vi "iRobot UART Open.vi"(9 "Baud Rate (BPS)":T1=enum."57600", 11 "UART port in":T2) -> (0 "error out":errorcluster, 3 "UART port out":T2)   [LabVIEW 2010]
doc: "Opens a UART session with an iRobot."
uses:
  UART Port Type.ctl
  Command/Command Controls/iRobot Baud.ctl
  <vilib>/Instr/_visa.llb/VISA Configure Serial Port (Instr).vi
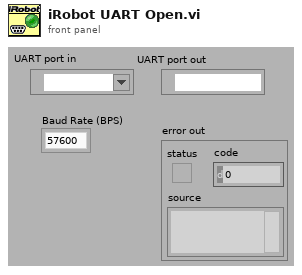
[diagram p1: front panel]
types:
  T1 = typedef "iRobot Baud.ctl" = enum8{"300", "600", "1200", "2400", "4800", "9600", "14400", "19200", "28800", "38400", "57600", "115200"}
  T2 = typedef "UART Port Type.ctl" = refnum<visa-resource-name>
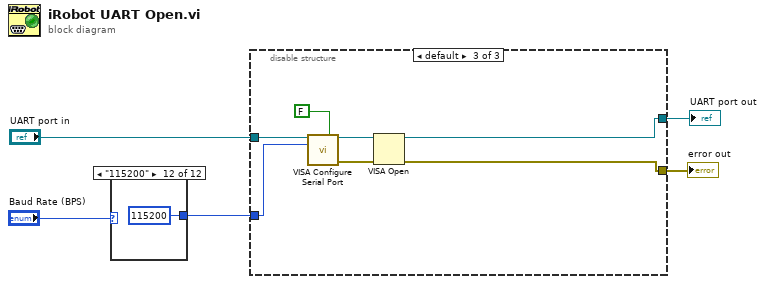
[diagram p0: block diagram]
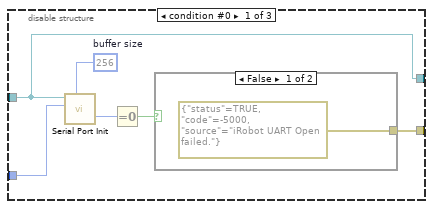
[diagram p2: hidden frame]
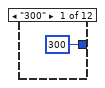
[diagram p5: hidden frame]
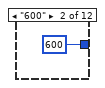
[diagram p6: hidden frame]
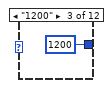
[diagram p7: hidden frame]
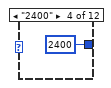
[diagram p8: hidden frame]
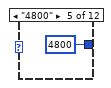
[diagram p9: hidden frame]
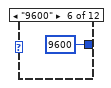
[diagram p10: hidden frame]
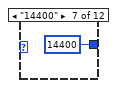
[diagram p11: hidden frame]
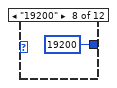
[diagram p12: hidden frame]
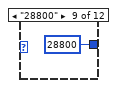
[diagram p13: hidden frame]
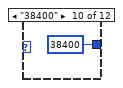
[diagram p14: hidden frame]
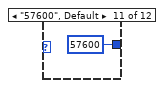
[diagram p15: hidden frame]
diagram:
  n1 = case shown="\"115200\"" "Baud Rate (BPS)" {
    tunnel: [u32 300 ("baud rate") u32 600 ("baud rate") u32 1200 ("baud rate") u32 2400 ("baud rate") u32 4800 ("baud rate") u32 9600 ("baud rate") u32 14400 ("baud rate") u32 19200 ("baud rate") u32 28800 ("baud rate") u32 38400 ("baud rate") u32 57600 ("baud rate") u32 115200 ("baud rate")] -> w3
    frame "300" {
    }
    frame "600" {
    }
    frame "1200" {
    }
    frame "2400" {
    }
    frame "4800" {
    }
    frame "9600" {
    }
    frame "14400" {
    }
    frame "19200" {
    }
    frame "28800" {
    }
    frame "38400" {
    }
    frame "57600", Default {
    }
    frame "115200" {
    }
  }
  n2 = disable-structure shown="default" {
    disable-tunnel: "UART port in" -> [w18 _ w31]
    disable-tunnel: w3 -> [w23 _ w30]
    disable-tunnel: [w20 _ w25] -> w2
    disable-tunnel: [w18 _ w26] -> w1
    frame condition #0 {
      w19 = u16 256  # buffer size
      n3 = call <vilib>:"Serial Port Init.vi"("buffer size"=w19, "baud rate"=w23, "port number"=w18) -> ("error code"=w21:i32)  [unwired: 4 in]
      n4 = Equal To 0?(x=w21) -> (x = 0?=w22:bool)
      n5 = case shown="False" w22 {
        tunnel: [errorcluster {"status"=TRUE, "code"=-5000, "source"="iRobot UART Open failed."} ("error out") _] -> w20
        frame False {
        }
        frame True {
          # "No error"
        }
      }
    }
    frame condition #1 {
      # "To be deployed..."
    }
    frame condition #2 (active) {
      n6 = call-poly "VISA Configure Serial Port"("VISA resource name"=w31, "Enable Termination\nChar (T)"=FALSE ("Enable Termination\nChar (T)"), "baud rate (9600)"=w30) -> ("VISA resource name out"=w28:refnum<visa-resource-name>, "error out"=w27:errorcluster)  [unwired: 11 in]
      n7 = VISA Open(error in (no error)=w27, VISA resource name=w28) -> (VISA resource name=w26:refnum<visa-resource-name>, error out=w25:errorcluster)  [unwired: 3 in]
    }
  }
  "UART port out" <- w1
  "error out" <- w2
